vi "Analyze.vi"(6 "error in":errorcluster, 8 "n-channel data (2D DBL)":dbl[][](array[numeric])) -> (0 "error out":errorcluster, 2 "message":string)   [LabVIEW 2020]
uses:
  <vilib>/Analysis/5stat.llb/RMS (DBL).vi
  <vilib>/Analysis/NI_AALPro.lvlib
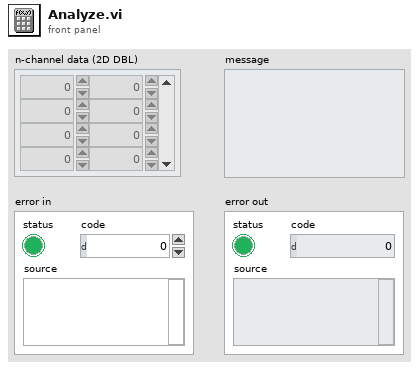
[diagram p1: front panel]
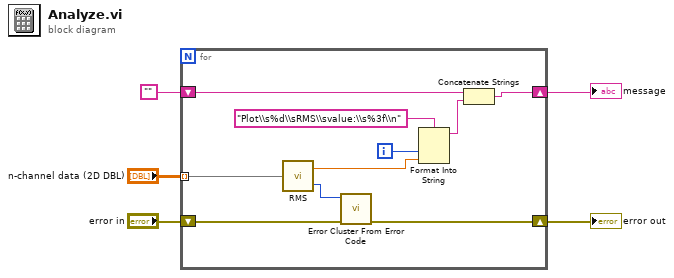
[diagram p0: block diagram]
diagram:
  n1 = for {
    tunnel: "n-channel data (2D DBL)" -> [w14] mode=indexing
    shift-right: [w8] -> w5
    shift-left: "" -> [w9]
    shift-right: [w15] -> w2
    shift-left: "error in" -> [w6]
    i -> [w13]
    n2 = call-poly <vilib>:"RMS.vi"("X"=w14) -> ("rms value"=w12:dbl, "error"=w7:i32)
    n3 = call <vilib>:"Error Cluster From Error Code.vi"("error in (no error)"=w6, "error code (0)"=w7) -> ("error out"=w15:errorcluster)  [unwired: 7 in]
    n4 = Format Into String(format string="Plot\\s%d\\sRMS\\svalue:\\s%3f\\n", w13, w12) -> (resulting string=w10:string)  [unwired: 2 in, 1 out]
    n5 = Concatenate Strings(w9, w10) -> (w8:string)
  }
  "message" <- w5
  "error out" <- w2
